vi "HW_GEN - Format Data Queue Name.vi"(10 "DevSN":string, 11 "DevName":string) -> (3 "Q Name":string)   [LabVIEW 2016]
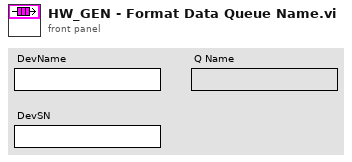
[diagram p1: front panel]
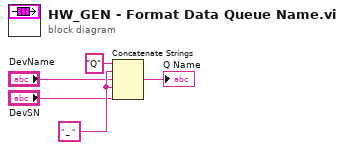
[diagram p0: block diagram]
diagram:
  w3 = " _ " ("string")
  n1 = Concatenate Strings("Q" ("string"), w3, "DevName", w3, "DevSN") -> (→"Q Name":string)
